vi "1553B_帧解析_v4.vi"(11 "数组":u8[](array[numeric])) -> (3 "输出簇":T1)   [LabVIEW 2012]
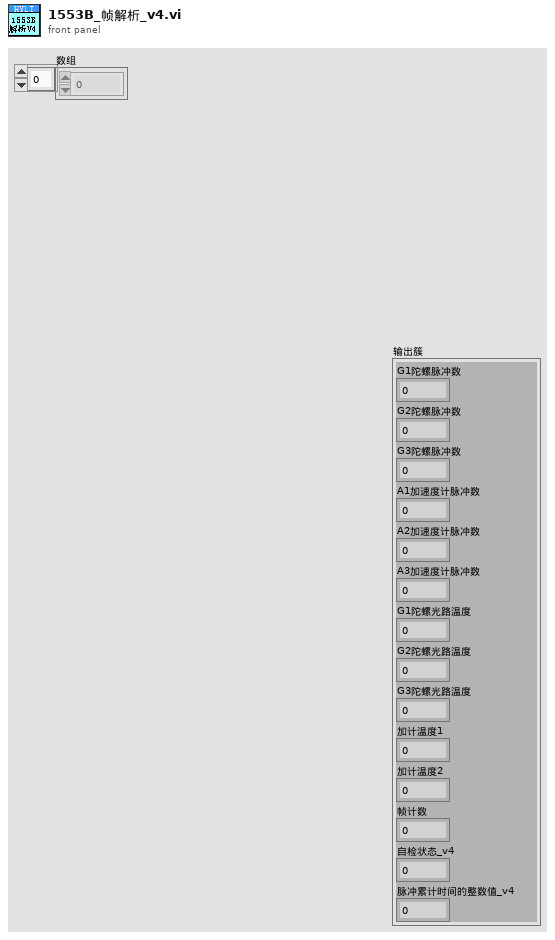
[diagram p1: front panel]
types:
  T1 = cluster{"G1陀螺脉冲数":i32, "G2陀螺脉冲数":i32, "G3陀螺脉冲数":i32, "A1加速度计脉冲数":i32, "A2加速度计脉冲数":i32, "A3加速度计脉冲数":i32, "G1陀螺光路温度":u8, "G2陀螺光路温度":u8, "G3陀螺光路温度":u8, "加计温度1":u8, "加计温度2":u8, "帧计数":u8, "自检状态_v4":u8, "脉冲累计时间的整数值_v4":u16}
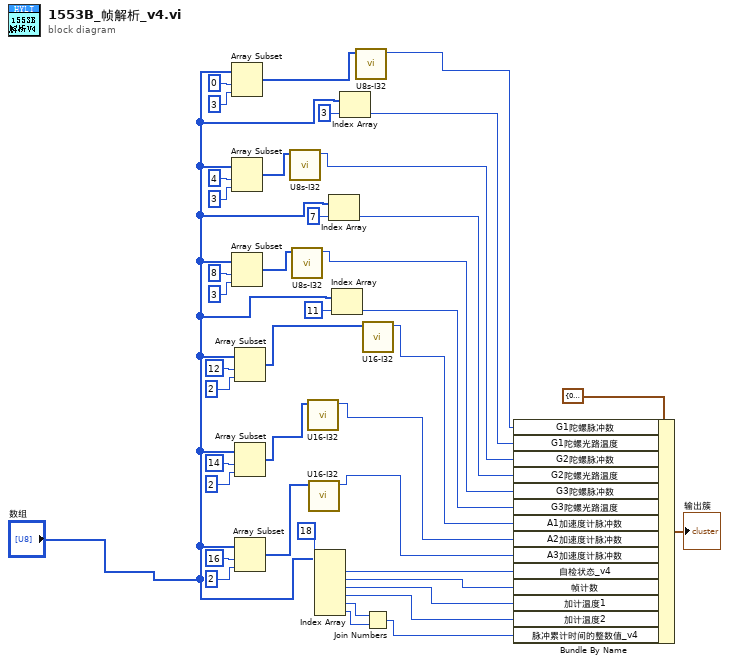
[diagram p0: block diagram]
diagram:
  n1 = Array Subset(array="数组", index=0 ("索引"), length=u8 3 ("新元素/子数组")) -> (w12:u8[])
  n2 = Array Subset(array="数组", index=4 ("索引"), length=u8 3 ("新元素/子数组")) -> (w10:u8[])
  n3 = Array Subset(array="数组", index=8 ("索引"), length=u8 3 ("新元素/子数组")) -> (w7:u8[])
  n4 = Array Subset(array="数组", index=12 ("索引"), length=u8 2 ("新元素/子数组")) -> (w6:u8[])
  n5 = Array Subset(array="数组", index=14 ("索引"), length=u8 2 ("新元素/子数组")) -> (w4:u8[])
  n6 = Array Subset(array="数组", index=16 ("索引"), length=u8 2 ("新元素/子数组")) -> (w2:u8[])
  n7 = call "U8s-I32.vi"("数组"=w10) -> ("I32转换"=w9:i32)  [unwired: 10 in]
  n8 = call "U8s-I32.vi"("数组"=w7) -> ("I32转换"=w8:i32)  [unwired: 10 in]
  n9 = call "U16-I32.vi"("数组"=w4) -> ("I32转换"=w3:i16)  [unwired: 10 in]
  n10 = call "U16-I32.vi"("数组"=w2) -> ("I32转换"=w1:i16)  [unwired: 10 in]
  n11 = Index Array(array="数组", index #1=18 ("索引")) -> (element #1=w28:u8, element #2=w27:u8, element #3=w26:u8, element #4=w25:u8, element #5=w23:u8, element #6=w22:u8)  [unwired: 5 in]
  n12 = Index Array(array="数组", index=7 ("索引")) -> (element=w17:u8)
  n13 = Index Array(array="数组", index=11 ("索引")) -> (element=w15:u8)
  n14 = Index Array(array="数组", index=3 ("索引")) -> (element=w19:u8)
  n15 = call "U8s-I32.vi"("数组"=w12) -> ("I32转换"=w11:i32)  [unwired: 10 in]
  n16 = call "U16-I32.vi"("数组"=w6) -> ("I32转换"=w5:i16)  [unwired: 10 in]
  n17 = Join Numbers(hi=w23, lo=w22) -> ((hi.lo)=w21:u16)
  n18 = Bundle By Name(cluster=T1 {"G1陀螺脉冲数"=0, "G2陀螺脉冲数"=0, "G3陀螺脉冲数"=0, "A1加速度计脉冲数"=0, "A2加速度计脉冲数"=0, "A3加速度计脉冲数"=0, "G1陀螺光路温度"=0, "G2陀螺光路温度"=0, "G3陀螺光路温度"=0, "加计温度1"=0, "加计温度2"=0, "帧计数"=0, "自检状态_v4"=0, "脉冲累计时间的整数值_v4"=0} ("输入簇"), "G1陀螺脉冲数"=w11, "G1陀螺光路温度"=w19, "G2陀螺脉冲数"=w9, "G2陀螺光路温度"=w17, "G3陀螺脉冲数"=w8, "G3陀螺光路温度"=w15, "A1加速度计脉冲数"=w5, "A2加速度计脉冲数"=w3, "A3加速度计脉冲数"=w1, "自检状态_v4"=w28, "帧计数"=w27, "加计温度1"=w26, "加计温度2"=w25, "脉冲累计时间的整数值_v4"=w21) -> (→"输出簇":T1)
